vi "variantCtrlStepPath.vi"(4 "isRequired (T)":bool=TRUE, 6 "menu(get)":enum16{"get", "set"}(ring), 7 "procElement":variant, 8 "error in (no error)":errorcluster, 9 "File Pointer in":string, 11 "stepElement in":variant) -> (0 "error out":errorcluster, 1 "File Pointer out":string="mylog.txt", 3 "step\\element out":variant)   [LabVIEW 2024]
uses:
  controls/typeStepVarients.ctl
  variantCtrlString.vi
  proc.util.validateParamExist.vi
  <vilib>/Utility/error.llb/Clear Errors.vi
  util.error.create.vi
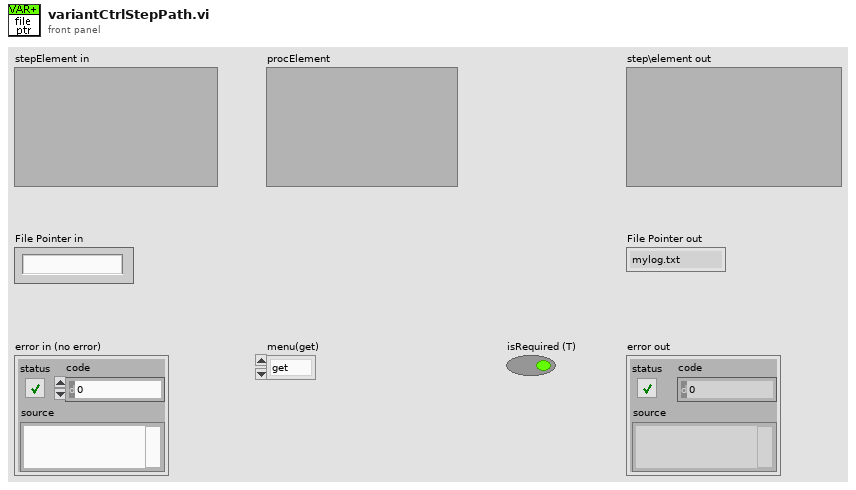
[diagram p1: front panel]
types:
  T1 = typedef "typeStepVarients.ctl" = enum16{"stepNameID", "stepFunction", "stepReport", "stepSetpoint", "stepPointer", "stepProcPointer", "stepIoPointer", "stepIoValue", "stepFilePointer", "stepMessage", "stepTimeString", "stepNumReg", "stepStrReg", "stepSeconds", "stepUnitDoseParams", "stepUnitIndex"}
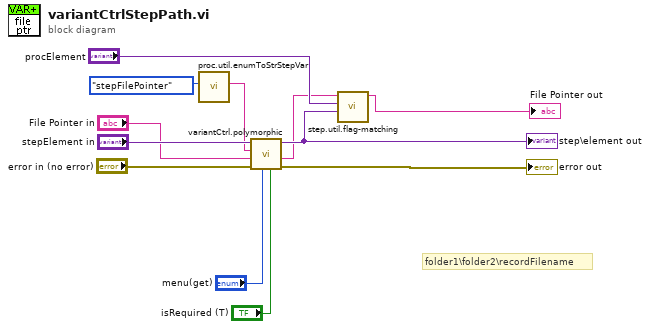
[diagram p0: block diagram]
diagram:
  # "folder1\\folder2\\recordFilename"
  n1 = call "proc.util.enumToStrStepVar.vi"("Step var"=typeStepVarients."stepFilePointer" ("proc var")) -> ("String"=w7:string)  [unwired: 10 in]
  n2 = call-poly "variantCtrl.polymorphic.vi"("isRequired (T)"="isRequired (T)", "menu in (get)"="menu(get)", "error in"="error in (no error)", "String Value"="File Pointer in", "name in"=w7, "Step in"="stepElement in") -> ("error out"=→"error out":errorcluster, "String Value"=w6:string, "Step out"=w8:variant)  [unwired: 2 in, 1 out]
  "step\\element out" <- w8
  n3 = call "step.util.flag-matching.vi"("stepElement"=w8, "procElement"="procElement", "$string in"=w6) -> ("formated string out"=→"File Pointer out":string)  [unwired: 8 in]
